vi "LVClass_WavefrontCorrectorSet GetGenericParameteBoolValue.vi"(0 "WavefrontCorrectorSet in":refnum<class "WavefrontCorrectorSet.lvclass">, 5 "parameter_name":string, 7 "DefaultFactorySet":bool, 11 "error in (no error)":errorcluster) -> (4 "WavefrontCorrectorSet out":refnum<class "WavefrontCorrectorSet.lvclass">, 6 "Value":bool, 15 "error out":errorcluster)   [LabVIEW 2020, in "WavefrontCorrectorSet.lvclass"]
doc: "WavefrontCorrector parameter default value getter for parameter of type\nboolean.\n\n--------------------------------------------------------------------------------\n\n<B>wavefrontcorrector_setIn </B> : WavefrontCorrectorSet object.\n<B>wavefrontcorrector_setOut </B> : WavefrontCorrectorSet object.\n<B>parameter_name </B> : Parameter name.\n<B>default_value </B> : Parameter default value.\n<B>ErrorIn </B> : Error\n<B>ErrorOut </B> : Error\n\n--------------------------------------------------------------------------------"
uses:
  WavefrontCorrectorSet.lvclass
  WavefrontCorrectorSet.lvclass/WavefrontCorrectorSet.ctl
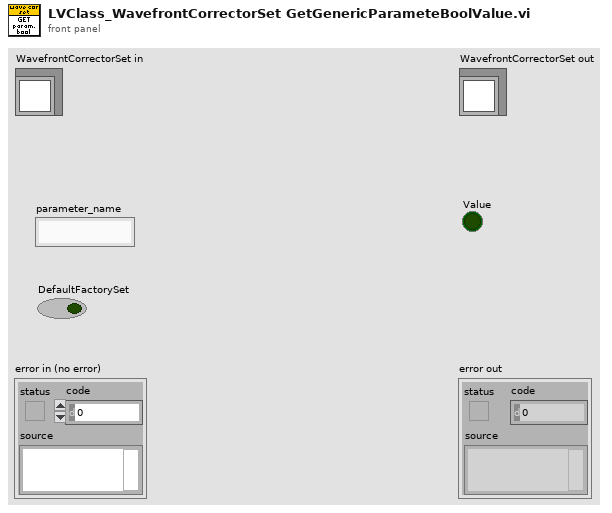
[diagram p1: front panel]
types:
  T1 = typedef "ClassID.ctl" = i64
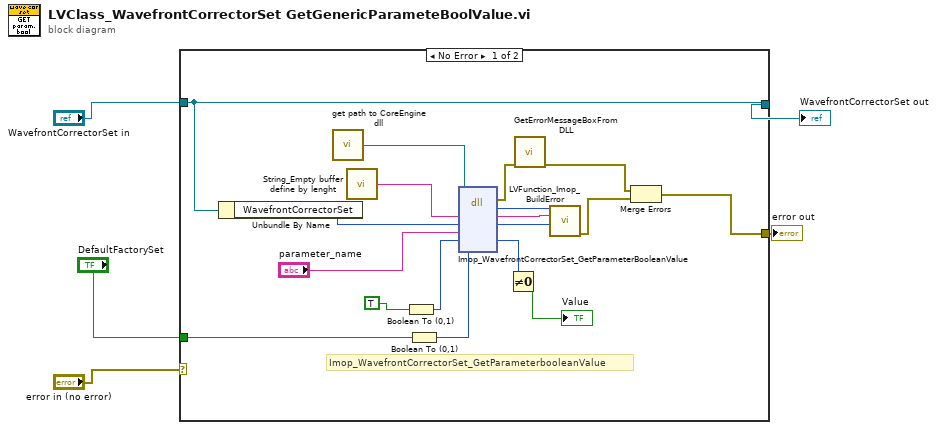
[diagram p0: block diagram]
diagram:
  n1 = case shown="No Error" "error in (no error)" {
    selector: "error in (no error)" -> [_ w24]
    tunnel: "WavefrontCorrectorSet in" -> [w13 w25]
    tunnel: [w13 w25] -> w3
    tunnel: [w11 w24] -> w2
    tunnel: "DefaultFactorySet" -> [w8 _]
    frame No Error {
      # "Imop_WavefrontCorrectorSet_GetParameterbooleanValue"
      n2 = Unbundle By Name(w13) -> ("WavefrontCorrectorSet"=w12:T1)
      n3 = call "get path to CoreEngine dll.vi"() -> ("path to wavekit library"=w19:path)  [unwired: 14 in, 1 out]
      n4 = call "String_Empty buffer define by lenght.vi"() -> ("Empty buffer"=w21:string)  [unwired: 1 in]
      n5 = Boolean To (0,1)(Boolean=TRUE) -> (0, 1=w16:i16)
      n6 = Boolean To (0,1)(Boolean=w8) -> (0, 1=w7:i16)
      n7 = dll-call lib="D:/soft/HASO_v3/SVN_trunk/ImOpCoreEngine4_LV2011/DLLs/c_interface_vc100.dll" fn="Imop_WavefrontCorrectorSet_GetParameterBooleanValue"(path in=w19, "message"=w21, "objet"=w12, "parameter_name"="parameter_name", "Value"=w16, "DefaultFactorySet"=w7) -> (error out=w18:errorcluster, "return type"=w23:i32, "message"=w22:string, "objet"=w6:i64, "Value"=w15:u8)  [unwired: 4 in, 1 out]
      n8 = Not Equal To 0?(x=w15) -> (x != 0?=→"Value":bool)
      n9 = call "GetErrorMessageBoxFromDLL.vi"("error IN"=w18) -> ("error OUT"=w10:errorcluster)  [unwired: 10 in]
      n10 = call "LVFunction_Imop_BuildError.vi"("code"=w23, "String to Prepend to source (\"\")"=w22, "Adresse"=w6) -> ("error out"=w9:errorcluster)  [unwired: 12 in]
      n11 = Merge Errors(w10, w9) -> (w11:errorcluster)
    }
    frame Error {
    }
  }
  "error out" <- w2
  "WavefrontCorrectorSet out" <- w3
